vi "cast u-64-0 to u64.vi"(11 "fixedpoint_i":fxp<+,64,0>) -> (3 "aifxp":u64)   [LabVIEW 2020, in "fixedpoint-cast.lvlib"]
uses:
  fixedpoint-cast.lvlib
  <vilib>/rvi/IPIntegrationNode/IPINode_Typedef/niFpgaIPINodeSupportedFamilies.ctl
  <vilib>/rvi/IPIntegrationNode/IPINode_Utilities/niFpgaIPINodeSimCore.vi
  <vilib>/rvi/IPIntegrationNode/IPINode_Xnode/niFpgaIPINode.xnode
  fixedpoint_vhdl/src/cast_u_dash_64_dash_0_to_u64SimFiles/xsim.dir/fixedpoint_to_u64/xsimkE178A56B595B48B8AB91732B5607448B.dll
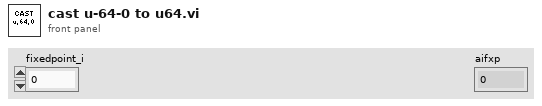
[diagram p1: front panel]
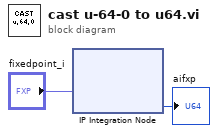
[diagram p0: block diagram]
diagram:
  n1 = xnode "IP Integration Node"("fixedpoint_i"="fixedpoint_i") -> ("u64_o"=→"aifxp":u64)
